vi "Deploy-Step-390-CustomizeSetupScript.vi"(0 "Deployment Engine":refnum<class "Deploy-DeploymentEngine.lvclass">, 11 "error in":errorcluster) -> (15 "error out":errorcluster)   [LabVIEW 2012]
uses:
  <resource>/Framework/Providers/Wirebird Labs LLC/Deploy/Support/Deployment Engine Class/Deploy-DeploymentEngine.lvclass
panel:
  # "Inputs"
  # "Outputs"
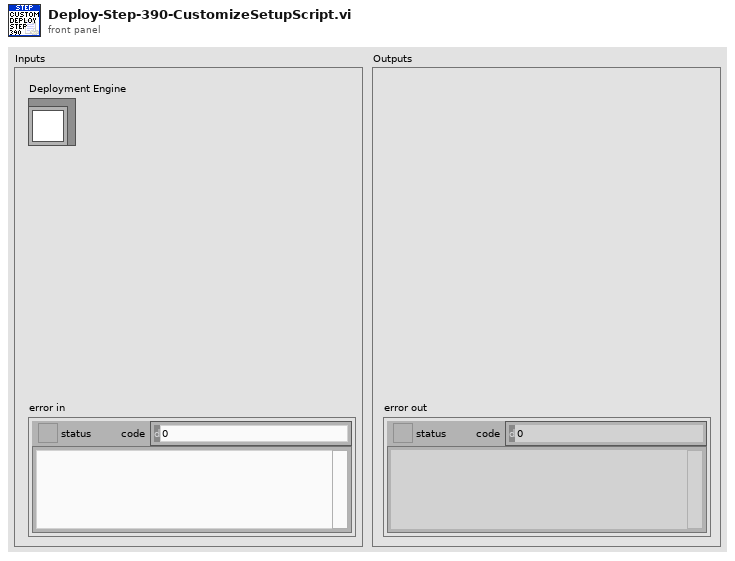
[diagram p1: front panel]
types:
  T1 = cluster{"Search for (Regular Expression)":string, "Replace with":string}[]
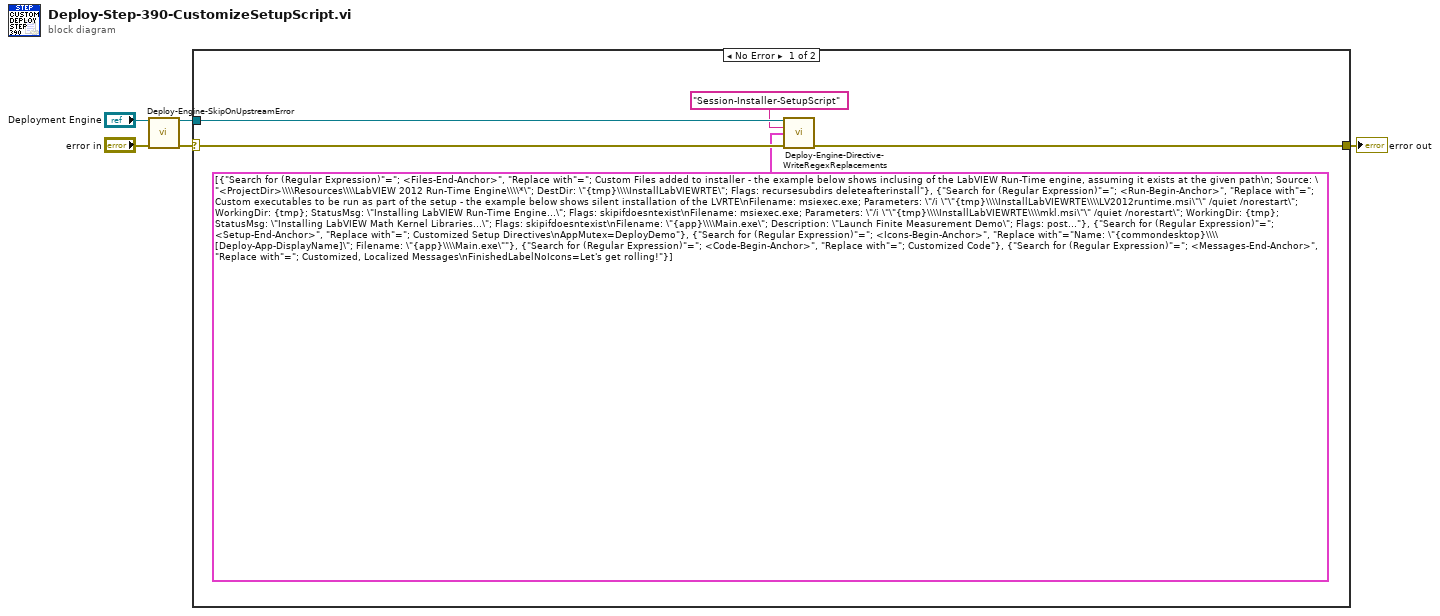
[diagram p0: block diagram]
diagram:
  n1 = call <resource>:"Deploy-Engine-SkipOnUpstreamError.vi"("Engine"="Deployment Engine", "error in"="error in") -> ("Engine out"=w2:refnum<class "Deploy-DeploymentEngine.lvclass">, "error out"=w1:errorcluster)  [unwired: 12 in]
  n2 = case shown="No Error" w1 {
    selector: w1 -> [w9 w11]
    tunnel: [w7 w11] -> w3
    tunnel: w2 -> [w10 _]
    frame No Error {
      n3 = call <resource>:"Deploy-Engine-Directive-WriteRegexReplacements.vi"("Engine"=w10, "Directive"="Session-Installer-SetupScript" ("Property Name"), "Value Replacements"=T1 [{"Search for (Regular Expression)"="; <Files-End-Anchor>", "Replace with"="; Custom Files added to installer - the example below shows inclusing of the LabVIEW Run-Time engine, assuming it exists at the given path\n; Source: \"<ProjectDir>\\\\Resources\\\\LabVIEW 2012 Run-Time Engine\\\\*\"; DestDir: \"{tmp}\\\\InstallLabVIEWRTE\"; Flags: recursesubdirs deleteafterinstall"}, {"Search for (Regular Expression)"="; <Run-Begin-Anchor>", "Replace with"="; Custom executables to be run as part of the setup - the example below shows silent installation of the LVRTE\nFilename: msiexec.exe; Parameters: \"/i \"\"{tmp}\\\\InstallLabVIEWRTE\\\\LV2012runtime.msi\"\" /quiet /norestart\"; WorkingDir: {tmp}; StatusMsg: \"Installing LabVIEW Run-Time Engine...\"; Flags: skipifdoesntexist\nFilename: msiexec.exe; Parameters: \"/i \"\"{tmp}\\\\InstallLabVIEWRTE\\\\mkl.msi\"\" /quiet /norestart\"; WorkingDir: {tmp}; StatusMsg: \"Installing LabVIEW Math Kernel Libraries...\"; Flags: skipifdoesntexist\nFilename: \"{app}\\\\Main.exe\"; Description: \"Launch Finite Measurement Demo\"; Flags: postinstall nowait\n"}, {"Search for (Regular Expression)"="; <Setup-End-Anchor>", "Replace with"="; Customized Setup Directives\nAppMutex=DeployDemo"}, {"Search for (Regular Expression)"="; <Icons-Begin-Anchor>", "Replace with"="Name: \"{commondesktop}\\\\[Deploy-App-DisplayName]\"; Filename: \"{app}\\\\Main.exe\""}, {"Search for (Regular Expression)"="; <Code-Begin-Anchor>", "Replace with"="; Customized Code"}, {"Search for (Regular Expression)"="; <Messages-End-Anchor>", "Replace with"="; Customized, Localized Messages\nFinishedLabelNoIcons=Let's get rolling!"}], "error in"=w9) -> ("error out"=w7:errorcluster)  [unwired: 10 in, 1 out]
    }
    frame Error {
    }
  }
  "error out" <- w3
